vi "Disconnect.vi"(8 "error in":errorcluster, 11 "connection info":T1) -> (0 "error out":errorcluster)   [LabVIEW 2015, in "Diagnostics Host Automation API.lvlib"]
uses:
  Diagnostics Host Automation API.lvlib
  <vilib>/NI/STM/TCP/TCP Connection Info.ctl
  <vilib>/NI/STM/SubVIs/MetaDataElement.ctl
  <vilib>/NI/STM/TCP/Get Connection Reference (TCP).vi
  <vilib>/NI/STM/NI STM.lvlib
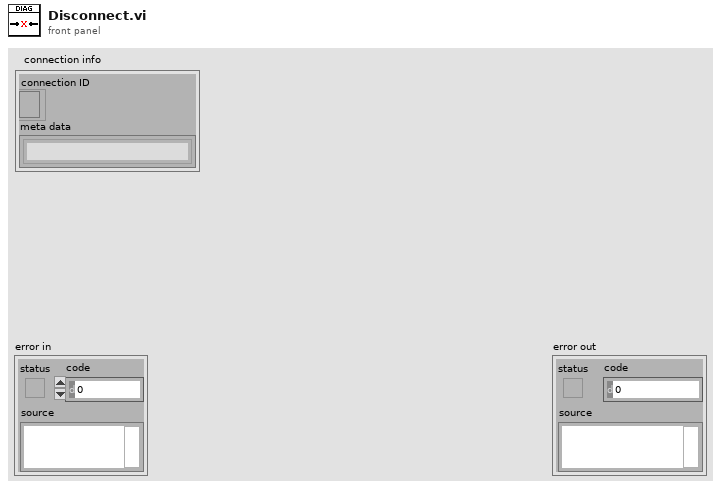
[diagram p1: front panel]
types:
  T1 = typedef "NI STM.lvlib/TCP Connection Info.ctl" = cluster{"connection ID":refnum<k5>, "meta data":T2[]}
  T2 = typedef "NI STM.lvlib/MetaDataElement.ctl" = string
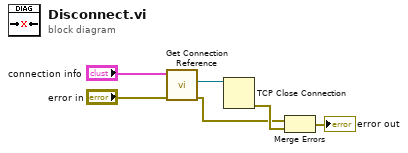
[diagram p0: block diagram]
diagram:
  n1 = call-poly <vilib>:"Get Connection Reference.vi"("error in"="error in", "connection info in"="connection info") -> ("error out"=w2:errorcluster, "connection ID out"=w6:refnum<k5>)  [unwired: 7 in, 1 out]
  n2 = TCP Close Connection(connection ID=w6) -> (error out=w3:errorcluster)  [unwired: 2 in, 1 out]
  n3 = Merge Errors(w2, w3) -> (→"error out":errorcluster)
